vi "Name.vi"(8 "error in (no error)":errorcluster, 11 "Runnable in":refnum<class "Parameter.lvclass">) -> (0 "error out":errorcluster, 2 "Name":string, 3 "Runnable out":refnum<class "Parameter.lvclass">)   [LabVIEW 2020, in "Parameter.lvclass"]
uses:
  Parameter.lvclass
  Parameter.lvclass/Parameter.ctl
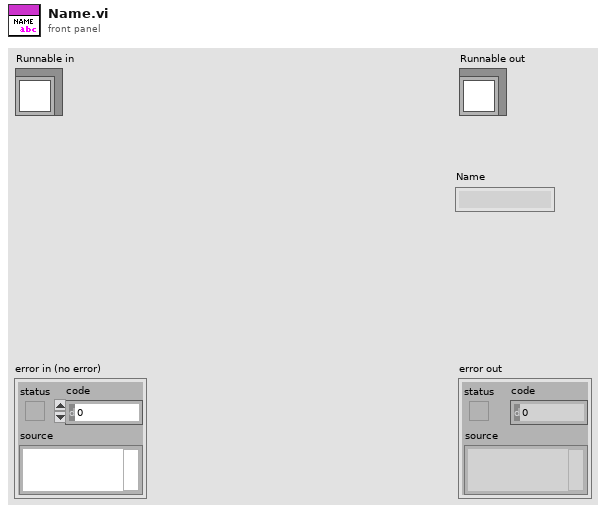
[diagram p1: front panel]
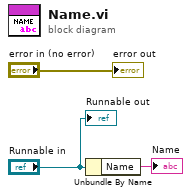
[diagram p0: block diagram]
diagram:
  n1 = Unbundle By Name("Runnable in") -> ("Name"=→"Name":string)
  "error out" <- "error in (no error)"
  "Runnable out" <- "Runnable in"
